vi "WPI_CANTalonSRX_SendMotionProfile.vi"(0 "CAN Talon SRX Ref":T2={"DeviceStatus"={"status"=FALSE, "code"=0, "source"=""}, "Type"=enum."PWM", "PWM"={"PWM Channel"=enum."PWM 1", "DeadBand"={"Name"="", "maxPositivePwm"=0, "minPositivePwm"=0, "centerPwm"=0, "maxNegativePwm"=0, "minNegativePwm"=0, "angularRange"=0}}, "CAN"={"Device Number"=0, "SetOutput VI Ref"=variant(enum8{"Percent VBus", "Current", "Speed", "Position", "Voltage"} enum."Percent VBus"), "GetOutput VI Ref"=variant(refnum<k1> refnum), "Enable VI Ref"=variant(dbl 12.0), "Disable VI Ref"=variant(enum8{"Percent VBus", "Speed", "Position", "Slave", "Unchanged / Invalid", "Voltage Compensation", "Current", "Motion Profile"} enum."Percent VBus"), "Data"=variant}, "Invert"=FALSE}, 5 "Clear":bool, 7 "Push":bool, 9 "New Point":T1, 11 "error in":errorcluster) -> (4 "CAN Talon SRX Ref Out":T2={"DeviceStatus"={"status"=FALSE, "code"=0, "source"=""}, "Type"=enum."PWM", "PWM"={"PWM Channel"=enum."PWM 1", "DeadBand"={"Name"="", "maxPositivePwm"=0, "minPositivePwm"=0, "centerPwm"=0, "maxNegativePwm"=0, "minNegativePwm"=0, "angularRange"=0}}, "CAN"={"Device Number"=0, "SetOutput VI Ref"=variant(enum8{"Percent VBus", "Current", "Speed", "Position", "Voltage"} enum."Percent VBus"), "GetOutput VI Ref"=variant(refnum<k1> refnum), "Enable VI Ref"=variant(dbl 12.0), "Disable VI Ref"=variant(enum8{"Percent VBus", "Speed", "Position", "Slave", "Unchanged / Invalid", "Voltage Compensation", "Current", "Motion Profile"} enum."Percent VBus"), "Data"=variant}, "Invert"=FALSE}, 8 "Count":u32, 10 "Ready For Next":bool, 15 "error out":errorcluster)   [LabVIEW 2016]
uses:
  <vilib>/Rock Robotics/WPI/MotorControl/WPI_MotorControlDeviceRef.ctl
  <vilib>/Rock Robotics/WPI/MotorControl/WPI_MotorControlType.ctl
  <vilib>/Rock Robotics/SystemInterfaces/DIO/FPGA_DIOPWMChannel.ctl
  <vilib>/Rock Robotics/WPI/PWM/WPI_PWMDeadband.ctl
  <vilib>/Rock Robotics/WPI/ThirdParty/CanMotor/TalonSRX/WPI_CANTalonSRX_MotionProfileTrajectoryPt.ctl
  <vilib>/Rock Robotics/WPI/ThirdParty/CanMotor/TalonSRX/WPI_CANTalonSRX_GlobalOps.ctl
  <vilib>/Rock Robotics/WPI/ThirdParty/CanMotor/TalonSRX/WPI_CANTalonSRX_GlobalStatus.ctl
  <vilib>/Rock Robotics/WPI/ThirdParty/CanMotor/TalonSRX/WPI_CANTalonSRX_MessageIDs.ctl
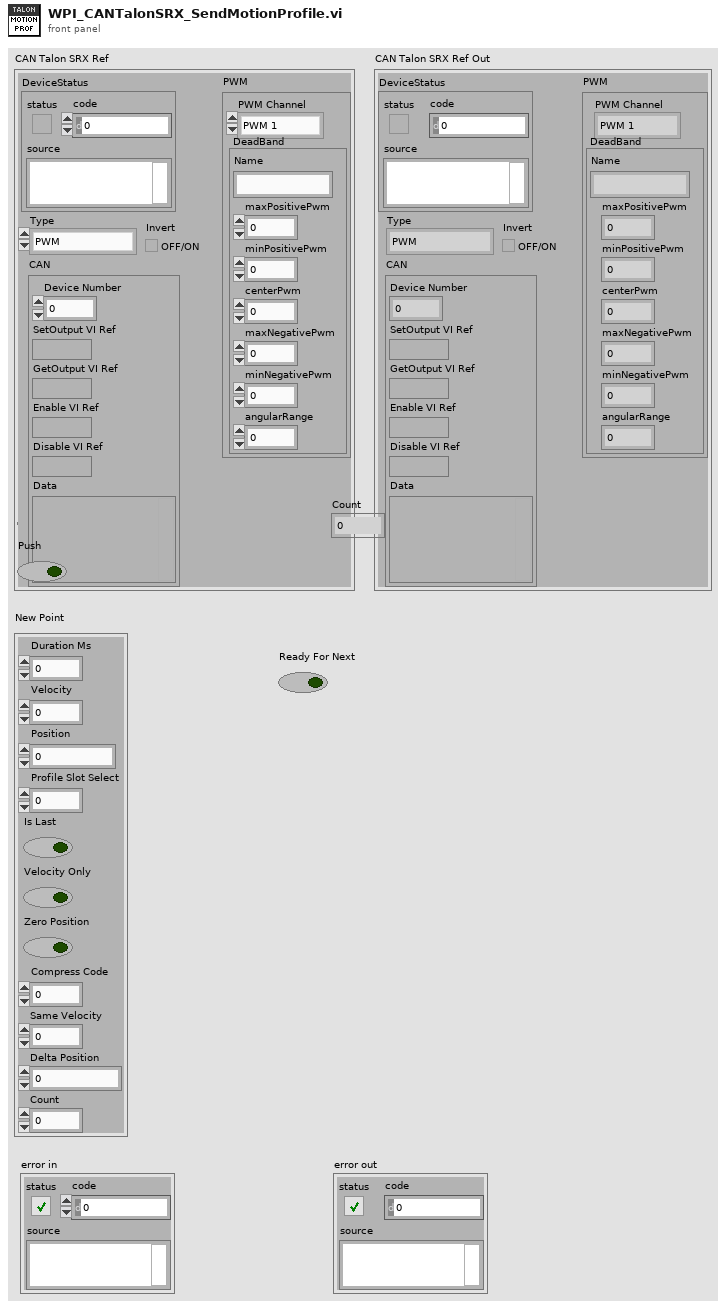
[diagram p1: front panel]
types:
  T1 = typedef "WPI_CANTalonSRX_MotionProfileTrajectoryPt.ctl" = cluster{"Duration Ms":u8, "Velocity":dbl, "Position":dbl, "Profile Slot Select":u8, "Is Last":bool, "Velocity Only":bool, "Zero Position":bool, "Compress Code":u8, "Same Velocity":i32, "Delta Position":i32, "Count":u8}
  T2 = typedef "WPI_MotorControlDeviceRef.ctl" = cluster{"DeviceStatus":errorcluster, "Type":T3, "PWM":cluster{"PWM Channel":T4, "DeadBand":T5}, "CAN":cluster{"Device Number":u8, "SetOutput VI Ref":variant, "GetOutput VI Ref":variant, "Enable VI Ref":variant, "Disable VI Ref":variant, "Data":variant}, "Invert":bool}
  T3 = typedef "WPI_MotorControlType.ctl" = enum16{"PWM", "CAN"}
  T4 = typedef "FPGA_DIOPWMChannel.ctl" = enum8{"PWM 0", "PWM 1", "PWM 2", "PWM 3", "PWM 4", "PWM 5", "PWM 6", "PWM 7", "PWM 8", "PWM 9", "PWM MXP 0", "PWM MXP 1", "PWM MXP 2", "PWM MXP 3", "PWM MXP 4", "PWM MXP 5", "PWM MXP 6", "PWM MXP 7", "PWM MXP 8", "PWM MXP 9", "Invalid"}
  T5 = typedef "WPI_PWMDeadband.ctl" = cluster{"Name":string, "maxPositivePwm":i32, "minPositivePwm":i32, "centerPwm":i32, "maxNegativePwm":i32, "minNegativePwm":i32, "angularRange":u16}
  T6 = typedef "WPI_CANTalonSRX_GlobalOps.ctl" = enum16{"Read For Send", "Write After Receive General", "Write After Receive Feedback", "Write After Receive Encoder", "Write After Receive Ain", "Write Error", "Get All", "Set Output", "Set Mode", "Set Master ID", "Set Brake Mode", "Set Reverse Feedback Sensor", "Set Reverse Closed Loop Output", "Set Override Limits", "Set Forward Limit Enabled", "Set Reverse Limit Enabled", "Set Feedback Select", "Set Profile Select", "Set Throttle Ramp Rate", "Disable", "Set Enc Codes Per Rev", "Set Num Pot Turns", "Set Control Frame Rate", "Enable Legacy Control", "Write After Receive Pulse Width", "Set Enable Frame Rate", "Write After Receive Motion Profile", "Set Motion Profile Flow Control", "Set Motion Profile Control Frame Rate"}
  T7 = typedef "WPI_CANTalonSRX_GlobalStatus.ctl" = cluster{"Applied Throttle":dbl, "Module Enabled":bool, "CAN Error":errorcluster, "Closed Loop Error":dbl, "Forward Limit Switch Closed":bool, "Reverse Limit Switch Closed":bool, "Sensor Position":dbl, "Sensor Velocity":dbl, "Current":dbl, "Sticky Fault - Over Temp":bool, "Sticky Fault - Under Voltage":bool, "Sticky Fault - Forward Limit":bool, "Sticky Fault - Reverse Limit":bool, "Sticky Fault - Forward Soft Limit":bool, "Sticky Fault - Reverse Soft Limit":bool, "Brake is Enabled":bool, "Encoder Position":dbl, "Encoder Velocity":dbl, "Encoder Index Count":dbl, "Encoder A Pin State":bool, "Encoder B Pin State":bool, "Encoder Index Pin State":bool, "Analog In":dbl, "Analog In Velocity":dbl, "Temperature (C)":dbl, "Battery Voltage":dbl, "Control 5 Is Supported":bool, "Current Profile Slot Select":dbl, "Pos Div 8":bool, "Vel Div 4":bool, "Pulse Width Position":i32, "Pulse Width Velocity":i32, "Pulse Width Rise To Rise (us)":i32, "Pulse Width Rise To Fall (us)":i32, "Mot Prof Active Is Under Run":bool, "Mot Prof Active Has Under Run":bool, "Mot Prof Active Is Last":bool, "Mot Prof Active Velocity Only":bool, "Mot Prof Active Is Valid":bool, "Mot Prof Buffer Is Full":bool, "Mot Prof Active Profile Slot Select":i32, "Mot Prof NextID":i32, "Mot Prof Count":i32, "Mot Prof Active Velocity":dbl, "Mot Prof Active Position":dbl, "Mot Prof Output Enable":i32}
  T8 = typedef "WPI_CANTalonSRX_MessageIDs.ctl" = u32
  T9 = typedef "WPI_CANTalonSRX_GlobalControl.ctl" = cluster{"Output":dbl, "Control Mode":T10, "Brake-Mode Override":T11, "Reverse Feedback Sensor":bool, "Reverse Closed-Loop Output":bool, "Override Limits":bool, "Forward Limit Enabled":bool, "Reverse Limit Enabled":bool, "Feedback Select":T12, "Profile Select":u8, "Master To Follow":u8, "Throttle Ramp Rate":u8, "Disabled":bool, "Encoder Codes Per Rev":u32, "Num Pot Turns":u32, "Control Frame Rate Ms":u8, "Use Control5 If Supported":bool, "Enable Frame Rate Ms":u8, "Motion Profile Flow Control":u8, "Motion Profile Control Frame Rate":u8, "Talon SRX Motion Profile Trajectory Point":T1}
  T10 = typedef "WPI_CANTalonSRX_APIControlMode.ctl" = enum8{"Percent VBus", "Speed", "Position", "Slave", "Unchanged / Invalid", "Voltage Compensation", "Current", "Motion Profile"}
  T11 = typedef "WPI_CANTalonSRX_BrakeOverride.ctl" = enum8{"No Override", "Override to Coast", "Override to Brake"}
  T12 = typedef "WPI_CANTalonSRX_FeedbackSelect.ctl" = u8
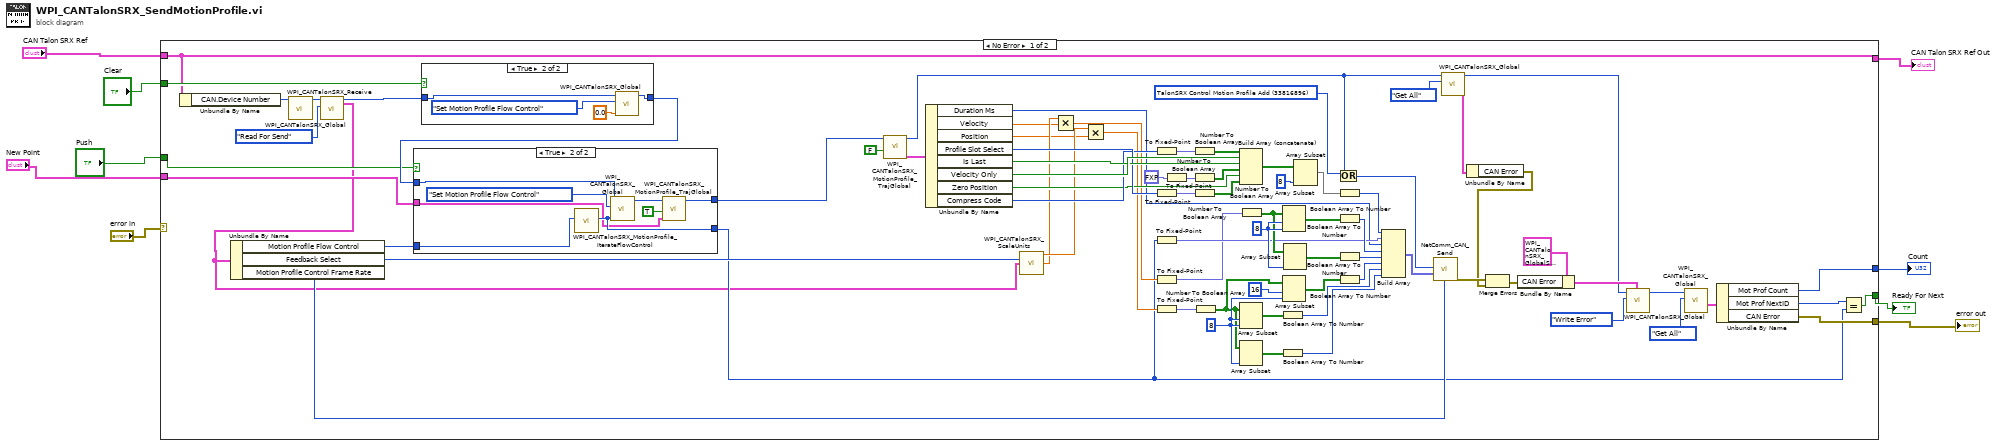
[diagram p0: block diagram]
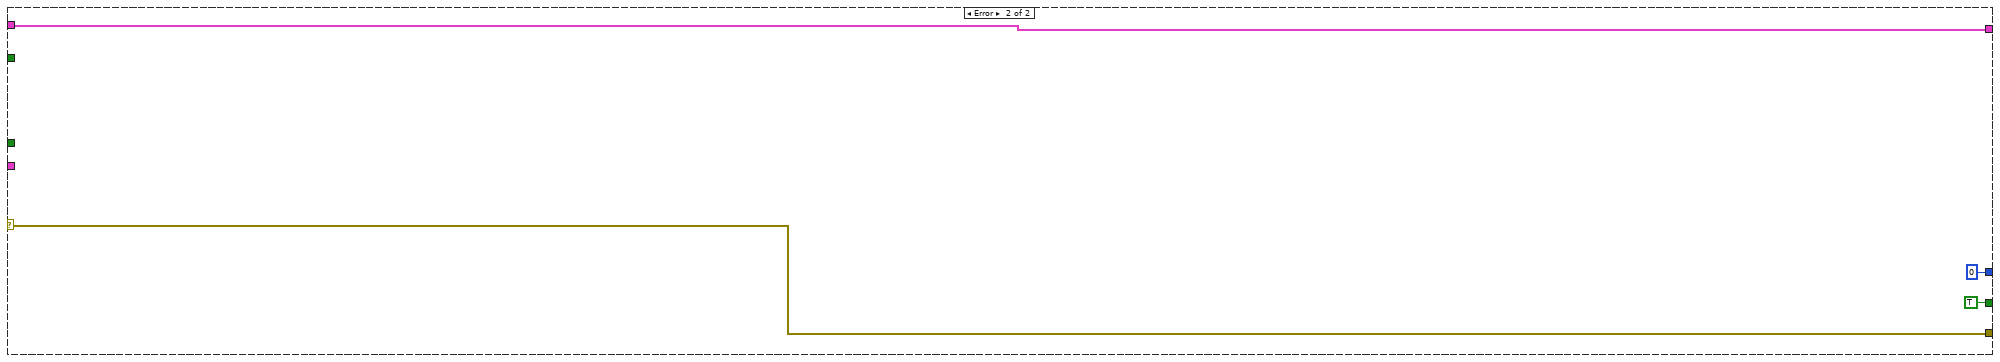
[diagram p4: hidden frame]
diagram:
  n1 = case shown="No Error" "error in" {
    selector: "error in" -> [_ w105]
    tunnel: [w77 w105] -> w8
    tunnel: "Clear" -> [w76 _]
    tunnel: "CAN Talon SRX Ref" -> [w75 w104]
    tunnel: [w75 w104] -> w5
    tunnel: [w72 TRUE] -> w4
    tunnel: "New Point" -> [w74 _]
    tunnel: "Push" -> [w73 _]
    tunnel: [w15 0 ("Mot Prof Count")] -> w1
    frame No Error {
      w12 = T8 33816896 items=["TalonSRX Control General 10ms"=33816576, "TalonSRX Control Rates Slow"=33816640, "TalonSRX Control ClearFlags Slow"=33816704, "TalonSRX Status General 10ms"=33821696, "TalonSRX Status Feedback 20ms"=33821760, "TalonSRX Status Enc 100ms"=33821824, "TalonSRX Status AinTempVbat 100ms"=33821888, "TalonSRX Status Startup Once"=33821952, "TalonSRX Status Debug"=33822080, "TalonSRX Config SetGainsSlot0 A"=33823808, "TalonSRX Config SetGainsSlot0 B"=33823872, "TalonSRX Config SetGainsSlot1 A"=33823936, "TalonSRX Config SetGainsSlot1 B"=33824000, "TalonSRX Config SetSoftLimits"=33824064, "TalonSRX Config WebControl"=33824128, "TalonSRX Param Request"=33822720, "TalonSRX Param Response"=33822784, "TalonSRX Param Set"=33822848, "TalonSRX Status PulseWidth"=33822144, "TalonSRX Status Motion Profile"=33822208, "TalonSRX Control General 5"=33816832, "TalonSRX Control Motion Profile Add"=33816896] ("Talon SRX Control Frame")
      w56 = 8 ("length")
      w67 = 8 ("length")
      n2 = Unbundle By Name(w75) -> ("CAN.Device Number"=w83:u8)
      n3 = call <vilib>:"WPI_CANTalonSRX_Receive.vi"("Device ID (0)"=w83) -> ("Device ID"=w84:u8)  [unwired: 10 in]
      n4 = call <vilib>:"WPI_CANTalonSRX_Global.vi"("Operation"=WPI_CANTalonSRX_GlobalOps."Read For Send", "Device ID (0)"=w84) -> ("Device ID Out"=w81:u8, "Read For Send"=w10:T9)  [unwired: 7 in, 1 out]
      n5 = Unbundle By Name(w10) -> ("Motion Profile Flow Control"=w14:u8, "Feedback Select"=w16:T12, "Motion Profile Control Frame Rate"=w25:u8)
      n6 = case shown="True" w76 {
        tunnel: w81 -> [w98 w101]
        tunnel: [w98 w100] -> w80
        frame False {
        }
        frame True {
          n7 = call <vilib>:"WPI_CANTalonSRX_Global.vi"("Set Number"=0.0, "Operation"=WPI_CANTalonSRX_GlobalOps."Set Motion Profile Flow Control", "Device ID (0)"=w101) -> ("Device ID Out"=w100:u8)  [unwired: 6 in, 2 out]
        }
      }
      n8 = case shown="True" w73 {
        tunnel: w74 -> [_ w93]
        tunnel: [w88 w97] -> w11
        tunnel: w80 -> [w89 w96]
        tunnel: [w89 w94] -> w79
        tunnel: w14 -> [w88 w91]
        frame False {
        }
        frame True {
          n9 = call <vilib>:"WPI_CANTalonSRX_MotionProfile_IterateFlowControl.vi"("Input"=w91) -> ("Output"=w97:i32)  [unwired: 10 in]
          n10 = call <vilib>:"WPI_CANTalonSRX_Global.vi"("Set Number"=w97, "Operation"=WPI_CANTalonSRX_GlobalOps."Set Motion Profile Flow Control", "Device ID (0)"=w96) -> ("Device ID Out"=w95:u8)  [unwired: 6 in, 2 out]
          n11 = call <vilib>:"WPI_CANTalonSRX_MotionProfile_TrajGlobal.vi"("Trajectory Point To Store"=w93, "Is Store"=TRUE, "Device ID (0)"=w95) -> ("Device ID Out"=w94:u8)  [unwired: 7 in, 1 out]
        }
      }
      n12 = call <vilib>:"WPI_CANTalonSRX_MotionProfile_TrajGlobal.vi"("Is Store"=FALSE, "Device ID (0)"=w79) -> ("Read For Send"=w24:T1, "Device ID Out"=w13:u8)  [unwired: 8 in]
      n13 = Unbundle By Name(w24) -> ("Duration Ms"=w33:u8, "Velocity"=w19:dbl, "Position"=w20:dbl, "Profile Slot Select"=w45:u8, "Is Last"=w49:bool, "Velocity Only"=w50:bool, "Zero Position"=w40:bool, "Compress Code"=w44:u8)
      n14 = call <vilib>:"WPI_CANTalonSRX_ScaleUnits.vi"("Feedback Scalar Select"=w16, "Read For Send"=w10) -> ("Position Scalar"=w22:dbl, "Velocity Scalar"=w21:dbl)  [unwired: 11 in, 1 out]
      n15 = Multiply(x=w19, y=w21) -> (x*y=w17:dbl)
      n16 = Multiply(x=w22, y=w20) -> (x*y=w18:dbl)
      n17 = To Fixed-Point(number=w11) -> (fixed-point=w34:fxp<+,4,4>)  [unwired: 1 in]
      n18 = To Fixed-Point(number=w44) -> (fixed-point=w47:fxp<+,2,2>)  [unwired: 1 in]
      n19 = To Fixed-Point(number=w45) -> (fixed-point=w46:fxp<+,1,1>)  [unwired: 1 in]
      n20 = To Fixed-Point(number=w17) -> (fixed-point=w31:fxp<+/-,16,16>)  [unwired: 1 in]
      n21 = To Fixed-Point(number=w18) -> (fixed-point=w32:fxp<+/-,24,24>)  [unwired: 1 in]
      n22 = To Fixed-Point(number=fxp<+/-,32,16> 0.0) -> (fixed-point=w48:fxp<+,2,2>)  [unwired: 1 in]
      n23 = Number To Boolean Array(number=w47) -> (Boolean array=w43:bool[])
      n24 = Number To Boolean Array(number=w48) -> (Boolean array=w41:bool[])
      n25 = Number To Boolean Array(number=w46) -> (Boolean array=w39:bool[])
      n26 = Number To Boolean Array(number=w32) -> (Boolean array=w57:bool[])
      n27 = Build Array (concatenate)(w43, w50, w49, w41, w40, w39) -> (w37:bool[])
      n28 = Array Subset(array=w57, index=w67, length=w67) -> (w60:bool[])
      n29 = Array Subset(array=w57, length=w67) -> (w58:bool[])  [unwired: 1 in]
      n30 = Number To Boolean Array(number=w31) -> (Boolean array=w53:bool[])
      n31 = Boolean Array To Number(Boolean array=w60) -> (number=w62:u32)
      n32 = Boolean Array To Number(Boolean array=w58) -> (number=w61:u32)
      n33 = Array Subset(array=w53, index=w56, length=w56) -> (w55:bool[])
      n34 = Array Subset(array=w57, index=16, length=w67) -> (w59:bool[])
      n35 = Array Subset(array=w53, length=w56) -> (w54:bool[])  [unwired: 1 in]
      n36 = Array Subset(array=w37, length=8) -> (w36:bool[])  [unwired: 1 in]
      n37 = Or(x=w12, y=w13) -> (x .or. y?=w30:T8)
      n38 = Boolean Array To Number(Boolean array=w36) -> (number=w35:u32)
      n39 = Boolean Array To Number(Boolean array=w55) -> (number=w51:u32)
      n40 = Boolean Array To Number(Boolean array=w54) -> (number=w52:u32)
      n41 = Boolean Array To Number(Boolean array=w59) -> (number=w63:u32)
      n42 = Build Array(w35, w34, w33, w51, w52, w63, w62, w61) -> (w71:fxp<+,32,32>[])
      n43 = call <vilib>:"NetComm_CAN_Send.vi"("Period (ms)"=w25, "Data"=w71, "Message ID"=w30) -> ("error out"=w65:errorcluster)  [unwired: 8 in]
      n44 = call <vilib>:"WPI_CANTalonSRX_Global.vi"("Operation"=WPI_CANTalonSRX_GlobalOps."Get All", "Device ID (0)"=w13) -> ("Get All"=w28:T7, "Device ID Out"=w26:u8)  [unwired: 7 in, 1 out]
      n45 = Unbundle By Name(w28) -> ("CAN Error"=w27:errorcluster)
      n46 = Merge Errors(w65, w27) -> (w64:errorcluster)
      n47 = Bundle By Name(cluster=T7 {"Applied Throttle"=0.0, "Module Enabled"=FALSE, "CAN Error"={"status"=FALSE, "code"=0, "source"=""}, "Closed Loop Error"=0.0, "Forward Limit Switch Closed"=FALSE, "Reverse Limit Switch Closed"=FALSE, "Sensor Position"=0.0, "Sensor Velocity"=0.0, "Current"=0.0, "Sticky Fault - Over Temp"=FALSE, "Sticky Fault - Under Voltage"=FALSE, "Sticky Fault - Forward Limit"=FALSE, "Sticky Fault - Reverse Limit"=FALSE, "Sticky Fault - Forward Soft Limit"=FALSE, "Sticky Fault - Reverse Soft Limit"=FALSE, "Brake is Enabled"=FALSE, "Encoder Position"=0.0, "Encoder Velocity"=0.0, "Encoder Index Count"=0.0, "Encoder A Pin State"=FALSE, "Encoder B Pin State"=FALSE, "Encoder Index Pin State"=FALSE, "Analog In"=0.0, "Analog In Velocity"=0.0, "Temperature (C)"=0.0, "Battery Voltage"=0.0, "Control 5 Is Supported"=FALSE, "Current Profile Slot Select"=0.0, "Pos Div 8"=FALSE, "Vel Div 4"=FALSE, "Pulse Width Position"=0, "Pulse Width Velocity"=0, "Pulse Width Rise To Rise (us)"=0, "Pulse Width Rise To Fall (us)"=0, "Mot Prof Active Is Under Run"=FALSE, "Mot Prof Active Has Under Run"=FALSE, "Mot Prof Active Is Last"=FALSE, "Mot Prof Active Velocity Only"=FALSE, "Mot Prof Active Is Valid"=FALSE, "Mot Prof Buffer Is Full"=FALSE, "Mot Prof Active Profile Slot Select"=0, "Mot Prof NextID"=0, "Mot Prof Count"=0, "Mot Prof Active Velocity"=0.0, "Mot Prof Active Position"=0.0, "Mot Prof Output Enable"=0} ("Write After Receive"), "CAN Error"=w64) -> (w68:T7)
      n48 = call <vilib>:"WPI_CANTalonSRX_Global.vi"("Write After Receive"=w68, "Operation"=WPI_CANTalonSRX_GlobalOps."Write Error", "Device ID (0)"=w26) -> ("Device ID Out"=w78:u8)  [unwired: 6 in, 2 out]
      n49 = call <vilib>:"WPI_CANTalonSRX_Global.vi"("Operation"=WPI_CANTalonSRX_GlobalOps."Get All", "Device ID (0)"=w78) -> ("Get All"=w85:T7)  [unwired: 7 in, 2 out]
      n50 = Unbundle By Name(w85) -> ("Mot Prof Count"=w15:i32, "Mot Prof NextID"=w82:i32, "CAN Error"=w77:errorcluster)
      n51 = Equal?(x=w82, y=w11) -> (x = y?=w72:bool)
    }
    frame Error {
    }
  }
  "error out" <- w8
  "CAN Talon SRX Ref Out" <- w5
  "Ready For Next" <- w4
  "Count" <- w1
